vi "GetSeparator2.vi"(8 "error in (no error)":errorcluster, 11 "TestTestResult in":refnum<class "_TextTestResult.lvclass">) -> (0 "error out":errorcluster, 2 "separator2":string, 3 "TestTestResult out":refnum<class "_TextTestResult.lvclass">)   [LabVIEW 2011, in "_TextTestResult.lvclass"]
uses:
  _TextTestResult.lvclass
  _TextTestResult.lvclass/_TextTestResult.ctl
panel:
  # "JKI VI Tester for LabVIEW\nhttp://jkisoft.com/vi-tester\nCopyright (C) 2007-2009, JKI <info@jkisoft.com>\nALL RIGHTS RESERVED"
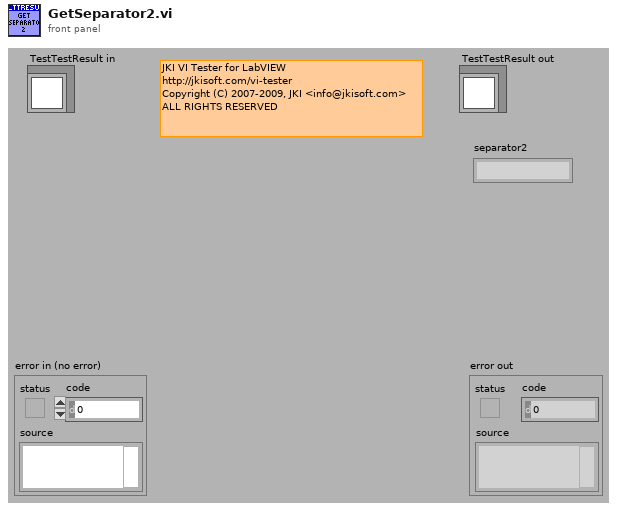
[diagram p1: front panel]
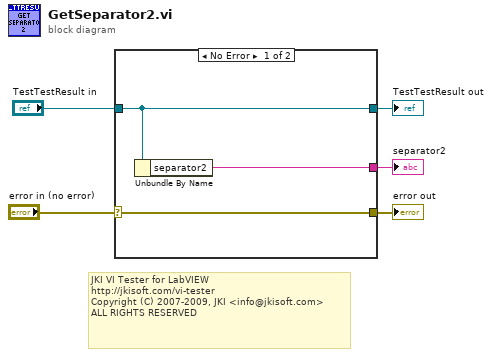
[diagram p0: block diagram]
diagram:
  # "JKI VI Tester for LabVIEW\nhttp://jkisoft.com/vi-tester\nCopyright (C) 2007-2009, JKI <info@jkisoft.com>\nALL RIGHTS RESERVED"
  n1 = case shown="No Error" "error in (no error)" {
    selector: "error in (no error)" -> [w7 w10]
    tunnel: [w7 w10] -> w4
    tunnel: [w6 w9] -> w2
    tunnel: "TestTestResult in" -> [w6 w9]
    tunnel: [w8 _] -> w1
    frame No Error {
      n2 = Unbundle By Name(w6) -> ("separator2"=w8:string)
    }
    frame Error {
    }
  }
  "error out" <- w4
  "TestTestResult out" <- w2
  "separator2" <- w1
